vi "ID Query.vi"(7 "error in (no error)":errorcluster, 10 "VISA resource name":refnum<visa-resource-name>) -> (0 "error out":errorcluster, 2 "read buffer":string, 3 "VISA resource name out":refnum<visa-resource-name>)   [LabVIEW 2025]
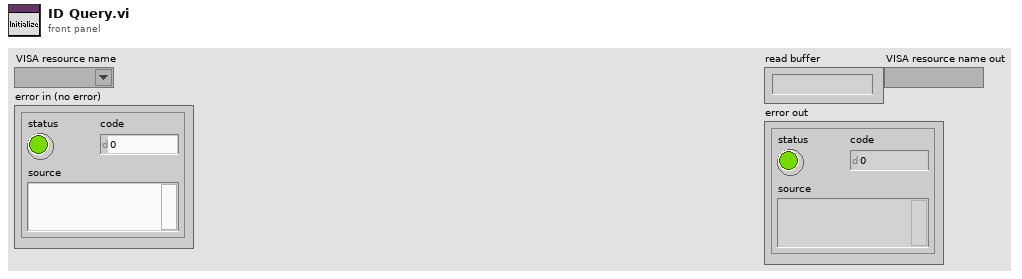
[diagram p1: front panel]
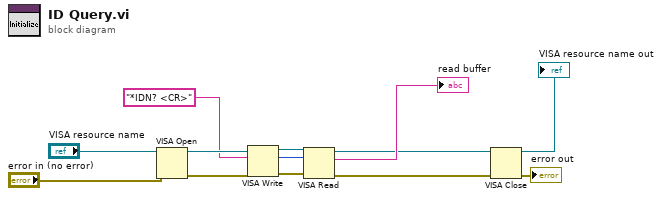
[diagram p0: block diagram]
diagram:
  n1 = VISA Open(error in (no error)="error in (no error)", VISA resource name="VISA resource name") -> (VISA resource name=w11:refnum<visa-resource-name>, error out=w12:errorcluster)  [unwired: 3 in]
  n2 = VISA Write(VISA resource name=w11, write buffer="*IDN? <CR>", error in (no error)=w12) -> (VISA resource name out=w7:refnum<visa-resource-name>, return count=w8:u32, error out=w9:errorcluster)
  n3 = VISA Read(VISA resource name=w7, byte count=w8, error in (no error)=w9) -> (VISA resource name out=w5:refnum<visa-resource-name>, read buffer=→"read buffer":string, error out=w4:errorcluster)  [unwired: 1 out]
  "VISA resource name out" <- w5
  n4 = VISA Close(VISA resource name=w5, error in (no error)=w4) -> (error out=→"error out":errorcluster)
